vi "Device Family Change.vi"(11 "Device ID":u32) -> (3 "New Family":bool)   [LabVIEW 2015]
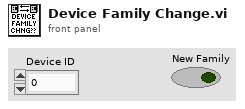
[diagram p1: front panel]
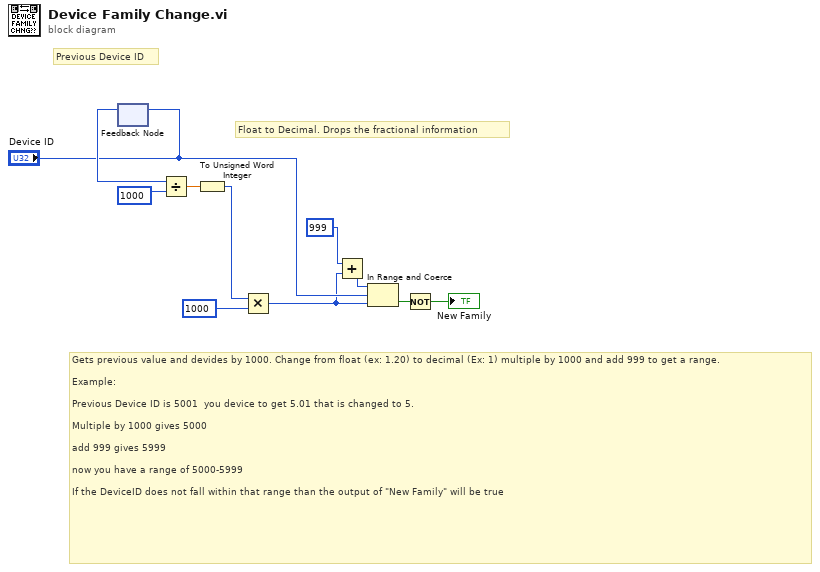
[diagram p0: block diagram]
diagram:
  # "Float to Decimal. Drops the fractional information"
  # "Previous Device ID"
  # "Gets previous value and devides by 1000. Change from float (ex: 1.20) to decimal (Ex: 1) multiple by 1000 and add 999 to get a range. \n\nExample:\n\nPrevious Device ID is 5001  you device to get 5.01 that is changed to 5.\n\nMultiple by 1000 gives 5000\n\nadd 999 gives 5999\n\nnow you have a range of 5000-5999\n\nIf the DeviceID does not fall within that range than the output of \"New Family\" will be true"
  n1 = feedback #1() -> (w11:u32)  [unwired: 1 in]
  n2 = feedback-in #1("Device ID") -> ()
  n3 = Divide(x=w11, y=u32 1000) -> (x/y=w9:dbl)
  n4 = To Unsigned Word Integer(number=w9) -> (unsigned 16bit integer=w7:u16)
  n5 = Multiply(x=w7, y=u16 1000) -> (x*y=w2:u16)
  n6 = Add(x=u16 999, y=w2) -> (x+y=w5:u16)
  n7 = In Range and Coerce(upper limit=w5, x="Device ID", lower limit=w2) -> (In Range?=w3:bool)  [unwired: 1 out]
  n8 = Not(x=w3) -> (.not. x?=→"New Family":bool)
